vi "Initialize Segmented Log.vi"(7 "Log File Specification":refnum<class "Log File Specification.lvclass">, 8 "error in (no error)":errorcluster, 9 "Max Instances (1)":i32=1, 11 "Segmented Log in":refnum<class "Segmented Log.lvclass">) -> (0 "error out":errorcluster, 3 "Segmented Log out":refnum<class "Segmented Log.lvclass">)   [LabVIEW 2015, in "Segmented Log.lvclass"]
uses:
  Segmented Log.lvclass
  Log File Specifications/Log File Specification/Log File Specification.lvclass
  Segmented Log Type.ctl
  Segmented Log.lvclass/Segmented Log.ctl
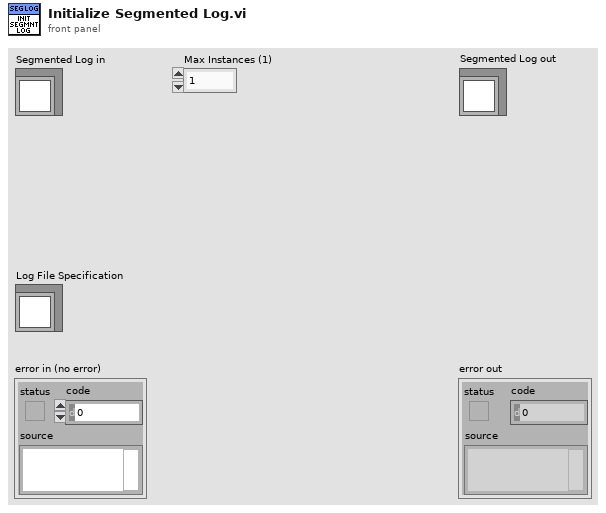
[diagram p1: front panel]
types:
  T1 = typedef "Segmented Log.lvclass/Segmented Log Type.ctl" = enum16{"No Limit", "Footprint", "Time"}
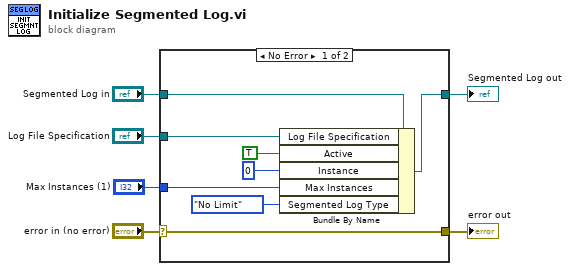
[diagram p0: block diagram]
diagram:
  n1 = case shown="No Error" "error in (no error)" {
    selector: "error in (no error)" -> [w8 w16]
    tunnel: [w8 w16] -> w5
    tunnel: [w9 w15] -> w4
    tunnel: "Log File Specification" -> [w12 _]
    tunnel: "Segmented Log in" -> [w11 w15]
    tunnel: "Max Instances (1)" -> [w10 _]
    frame No Error {
      n2 = Bundle By Name(cluster=w11, "Log File Specification"=w12, "Active"=TRUE, "Instance"=0, "Max Instances"=w10, "Segmented Log Type"=Segmented_Log_Type."No Limit") -> (w9:refnum<class "Segmented Log.lvclass">)
    }
    frame Error {
    }
  }
  "error out" <- w5
  "Segmented Log out" <- w4
